vi "Delete Column.vi"(8 "error in":errorcluster, 9 "Column path":string, 10 "Table Path":string, 11 "LV-Data.PG":refnum<class "LV-Data.PGSQL.lvclass">) -> (0 "error out":errorcluster, 3 "LV-Data.PG out":refnum<class "LV-Data.PGSQL.lvclass">)   [LabVIEW 2019, in "LV-Data.PGSQL.lvclass"]
uses:
  LV-Data.PGSQL.lvclass
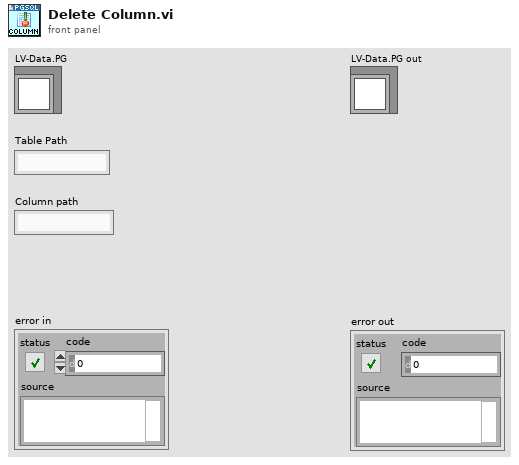
[diagram p1: front panel]
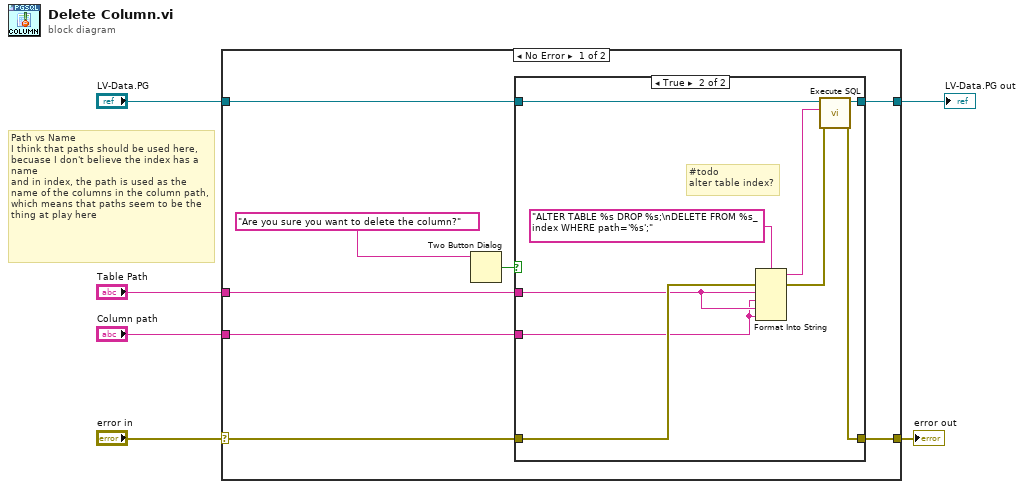
[diagram p0: block diagram]
diagram:
  # "Path vs Name\nI think that paths should be used here, becuase I don't believe the index has a name \nand in index, the path is used as the name of the columns in the column path, which means that paths seem to be the thing at play here"
  n1 = case shown="No Error" "error in" {
    selector: "error in" -> [w14 w27]
    tunnel: [w13 w27] -> w3
    tunnel: "Table Path" -> [w10 _]
    tunnel: "Column path" -> [w9 _]
    tunnel: "LV-Data.PG" -> [w12 w26]
    tunnel: [w11 w26] -> w1
    frame No Error {
      n2 = Two Button Dialog(message="Are you sure you want to delete the column?") -> (T button?=w8:bool)  [unwired: 2 in]
      n3 = case shown="True" w8 {
        tunnel: w14 -> [w15 w23]
        tunnel: [w15 w21] -> w13
        tunnel: w12 -> [w16 w20]
        tunnel: [w16 w19] -> w11
        tunnel: w10 -> [_ w18]
        tunnel: w9 -> [_ w17]
        frame False {
        }
        frame True {
          # "#todo\nalter table index?"
          n4 = Format Into String(format string="ALTER TABLE %s DROP %s;\nDELETE FROM %s_index WHERE path='%s';", error in=w23, w18, w17, w18, w17) -> (resulting string=w24:string, error out=w22:errorcluster)  [unwired: 1 in]
          n5 = call "Execute SQL.vi"("error in"=w22, "SQL"=w24, "LV-Data.PGSQL"=w20) -> ("error out"=w21:errorcluster, "LV-Data.PGSQL out"=w19:refnum<class "LV-Data.PGSQL.lvclass">)  [unwired: 5 in, 2 out]
        }
      }
    }
    frame Error {
    }
  }
  "error out" <- w3
  "LV-Data.PG out" <- w1
